vi "init.vi"(8 "error in":errorcluster, 11 "Analog_Input (in)":refnum<class "Analog_Input.lvclass">) -> (0 "error out":errorcluster, 3 "Analog_Input":refnum<class "Analog_Input.lvclass">)   [LabVIEW 2014, in "Analog_Input.lvclass"]
uses:
  Analog_Input.lvclass
  Analog_Input.lvclass/Analog_Input.ctl
  Globals.vi
  <vilib>/DAQmx/create/channels.llb/DAQmx Create Channel (AI-Voltage-Basic).vi
  <vilib>/DAQmx/configure/timing.llb/DAQmx Timing (Sample Clock).vi
  <vilib>/DAQmx/configure/trigger.llb/DAQmx Start Trigger (Digital Edge).vi
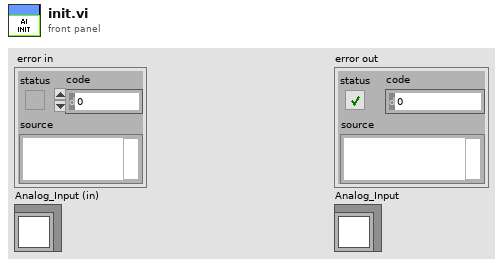
[diagram p1: front panel]
types:
  T1 = cluster{"Wait for start trigger?":bool, "source":tag, "edge":i32}
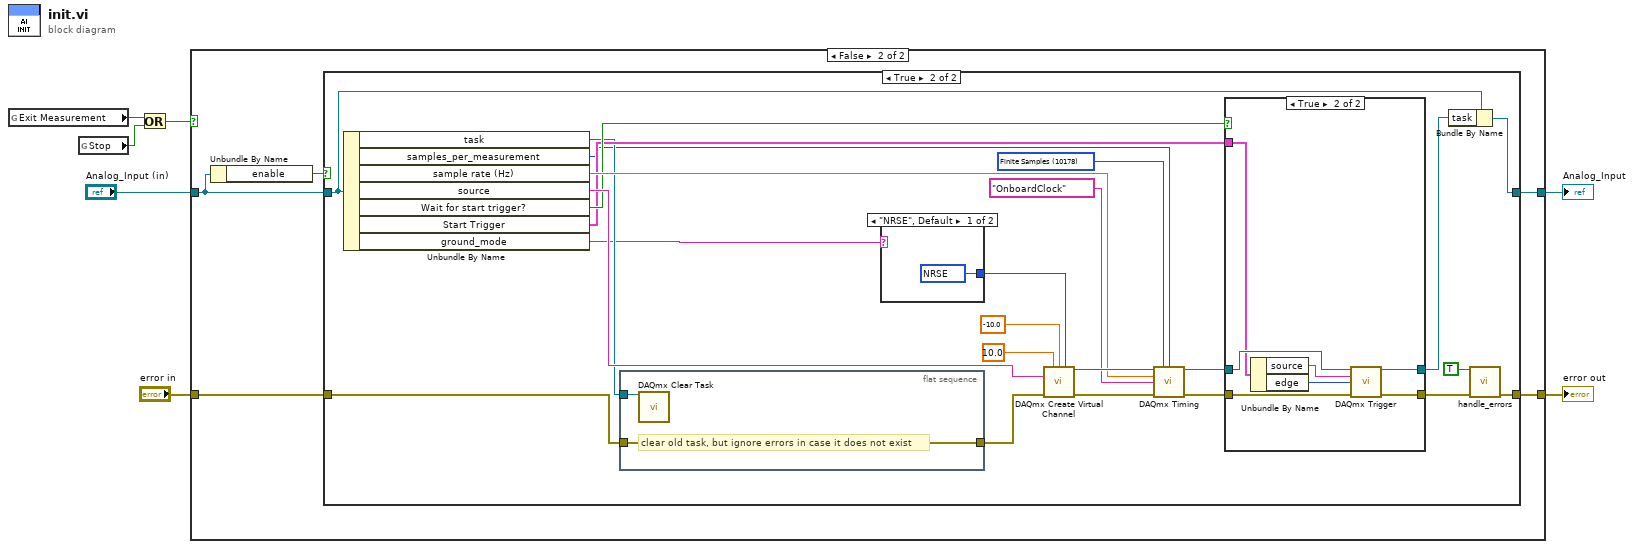
[diagram p0: block diagram]
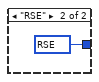
[diagram p4: hidden frame]
diagram:
  n1 = global read "Globals.vi" "Exit Measurement"() -> (w3:bool)
  n2 = global read "Globals.vi" "Stop"() -> (w2:bool)
  n3 = Or(x=w3, y=w2) -> (x .or. y?=w1:bool)
  n4 = case shown="False" w1 {
    tunnel: "error in" -> [w9 w14]
    tunnel: [w9 w13] -> w6
    tunnel: "Analog_Input (in)" -> [w8 w11]
    tunnel: [w8 w12] -> w4
    frame True {
    }
    frame False {
      n5 = Unbundle By Name(w11) -> ("enable"=w10:bool)
      n6 = case shown="True" w10 {
        tunnel: w14 -> [w16 w20]
        tunnel: [w16 w33] -> w13
        tunnel: w11 -> [w15 w31]
        tunnel: [w15 w32] -> w12
        frame False {
        }
        frame True {
          w37 = 10178 items=["Finite Samples"=10178, "Continuous Samples"=10123, "Hardware Timed Single Point"=12522] ("sample mode")
          n7 = Unbundle By Name(w31) -> ("task"=w21:refnum<k21>, "samples_per_measurement"=w18:i32, "sample rate (Hz)"=w30:dbl, "source"=w29:tag, "Wait for start trigger?"=w23:bool, "Start Trigger"=w22:T1, "ground_mode"=w17:string)
          n8 = flat-sequence {
            tunnel: w20 -> [w43]
            tunnel: [w43] -> w19
            tunnel: w21 -> [w44]
            frame #0 {
              # "clear old task, but ignore errors in case it does not exist"
              n9 = call <vilib>:"DAQmx Clear Task.vi"("task in"=w44) -> ()  [unwired: 14 in, 1 out]
            }
          }
          n10 = case shown="\"NRSE\", Default" w17 {
            tunnel: [w41 w42] -> w40
            frame "NRSE", Default {
              w41 = 10078 items=["default"=-1, "RSE"=10083, "NRSE"=10078, "Differential"=10106, "Pseudodifferential"=12529] ("input terminal configuration")
            }
            frame "RSE" {
              w42 = 10083 items=["default"=-1, "RSE"=10083, "NRSE"=10078, "Differential"=10106, "Pseudodifferential"=12529] ("input terminal configuration")
            }
          }
          n11 = call-poly <vilib>:"DAQmx Create Virtual Channel.vi"("maximum value"=10.0, "minimum value"=-10.0, "input terminal configuration"=w40, "physical channels"=w29, "error in"=w19) -> ("task out"=w39:refnum<k21>, "error out"=w38:errorcluster)  [unwired: 9 in]
          n12 = call-poly <vilib>:"DAQmx Timing.vi"("task/channels in"=w39, "sample mode"=w37, "samples per channel"=w18, "rate"=w30, "source"=tag "OnboardClock", "error in"=w38) -> ("task out"=w25:refnum<k21>, "error out"=w26:errorcluster)  [unwired: 8 in]
          n13 = case shown="True" w23 {
            tunnel: w25 -> [w46 w53]
            tunnel: [w46 w52] -> w24
            tunnel: w26 -> [w45 w51]
            tunnel: w22 -> [_ w50]
            tunnel: [w45 w47] -> w27
            frame False {
            }
            frame True {
              n14 = Unbundle By Name(w50) -> ("source"=w49:tag, "edge"=w48:i32)
              n15 = call-poly <vilib>:"DAQmx Trigger.vi"("task/channels in"=w53, "source"=w49, "edge"=w48, "error in"=w51) -> ("task out"=w52:refnum<k21>, "error out"=w47:errorcluster)  [unwired: 10 in]
            }
          }
          n16 = Bundle By Name(cluster=w31, "task"=w24) -> (w32:refnum<class "Analog_Input.lvclass">)
          n17 = call "handle_errors.vi"("Exit Operation"=TRUE, "error in (no error)"=w27) -> ("error out"=w33:errorcluster)  [unwired: 13 in]
        }
      }
    }
  }
  "error out" <- w6
  "Analog_Input" <- w4
